vi "interpolationSummer.vi"(7 "reset":bool, 8 "doStep":bool, 11 "upStep":fxp<+,22,0>) -> (3 "position":fxp<+,22,0>)   [LabVIEW 2016]
uses:
  <vilib>/rvi/FXPMathLib/FxpAdd/XNode/nifxpmath_Add.xnode
  <vilib>/rvi/FXPMathLib/sim/FxpSim.dll
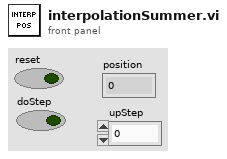
[diagram p1: front panel]
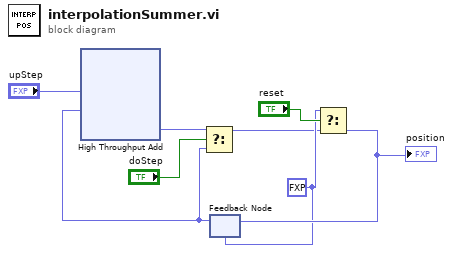
[diagram p0: block diagram]
diagram:
  w4 = fxp<+,16,0> 0.0 ("t")
  n1 = feedback #1(w4) -> (w2:fxp<+,22,0>)
  n2 = xnode ("High Throughput Add")("x"="upStep", "y"=w2) -> ("x+y"=w7:fxp<+,22,0>)
  n3 = Select(t=w7, s="doStep", f=w2) -> (s? t:f=w3:fxp<+,22,0>)
  n4 = Select(t=w4, s="reset", f=w3) -> (s? t:f=w6:fxp<+,22,0>)
  "position" <- w6
  n5 = feedback-in #1(w6) -> ()
